vi "Gyro to Heading.vi"(1 "Reset":bool, 2 "Angle In":dbl, 3 "GyroDevRef":T1) -> (0 "Heading":dbl)   [LabVIEW 2013]
uses:
  <vilib>/Rock Robotics/WPI/Gyro/WPI_GyroDevRef.ctl
  <vilib>/Rock Robotics/SystemInterfaces/Typedef/FPGA_TypedefAnalogModule.ctl
  <vilib>/Rock Robotics/SystemInterfaces/AI/FPGA_AIChannel.ctl
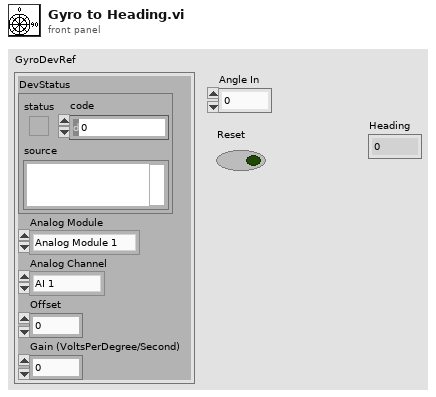
[diagram p1: front panel]
types:
  T1 = typedef "WPI_GyroDevRef.ctl" = cluster{"DevStatus":errorcluster, "Analog Module":T2, "Analog Channel":T3, "Offset":dbl, "Gain (VoltsPerDegree/Second)":dbl}
  T2 = typedef "FPGA_TypedefAnalogModule.ctl" = enum16{"Analog Module 1", "Analog Module 2"}
  T3 = typedef "FPGA_AIChannel.ctl" = enum8{"AI 1", "AI 2", "AI 3", "AI 4", "AI 5", "AI 6", "AI 7", "AI 8", "Invalid"}
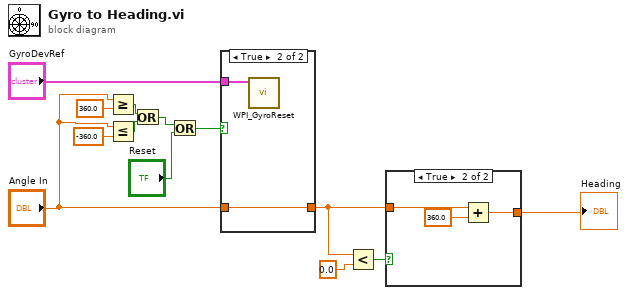
[diagram p0: block diagram]
diagram:
  n1 = Greater Or Equal?(x="Angle In", y=360.0) -> (x >= y?=w13:bool)
  n2 = Less Or Equal?(x="Angle In", y=-360.0) -> (x <= y?=w12:bool)
  n3 = Or(x=w13, y=w12) -> (x .or. y?=w7:bool)
  n4 = Or(x=w7, y="Reset") -> (x .or. y?=w6:bool)
  n5 = case shown="True" w6 {
    tunnel: "GyroDevRef" -> [_ w16]
    tunnel: [w14 w15] -> w2
    tunnel: "Angle In" -> [w14 w15]
    frame False {
    }
    frame True {
      n6 = call <vilib>:"WPI_GyroReset.vi"("GyroDevRef"=w16) -> ()  [unwired: 9 in, 2 out]
    }
  }
  n7 = Less?(x=w2, y=0.0) -> (x < y?=w3:bool)
  n8 = case shown="True" w3 {
    tunnel: [w17 w20] -> w4
    tunnel: w2 -> [w17 w19]
    frame False {
    }
    frame True {
      n9 = Add(x=w19, y=360.0) -> (x+y=w20:dbl)
    }
  }
  "Heading" <- w4
